vi "ColorDetect3.0_Display.vi"(4 "Fine Tune Upper":i32(slide)=119 scale=91.0..131.0, 5 "Max_radius":i32(slide)=50 scale=0.0..100.0, 6 "Fine Tune  Lower":i32(slide)=98 scale=85.0..125.0, 7 "Min_radius":i32(slide)=7 scale=0.0..100.0, 8 "error in (no error)":errorcluster, 10 "Upper (SV)":i32(slide)=223 scale=0.0..255.0, 11 "Lower (SV)":i32(slide)=58 scale=0.0..255.0) -> (0 "error out":errorcluster, 2 "XYR found":u32[][](array[numeric])=[[183, 192, 10]], 3 "found":i32=1)   [LabVIEW 2014, in "QwaveSys Raspberry Pi Library.lvlib"]
uses:
  QwaveSys Raspberry Pi Library.lvlib
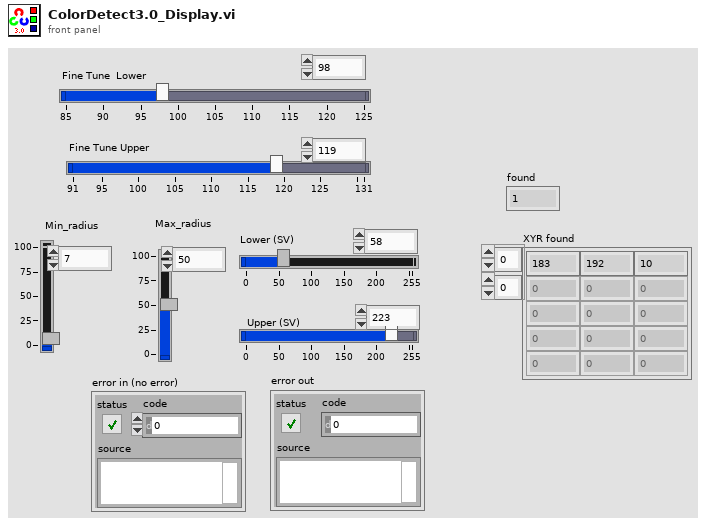
[diagram p1: front panel]
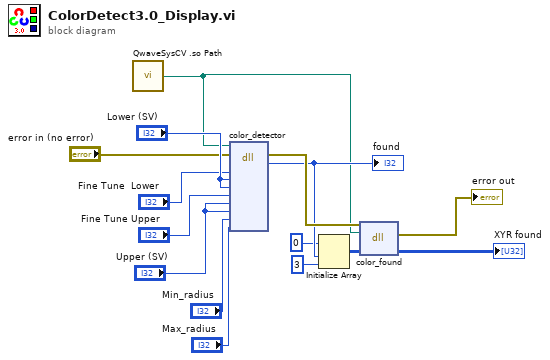
[diagram p0: block diagram]
diagram:
  n1 = call "QwaveSysCV .so Path.vi"() -> ("QwaveSys .so Path"=w5:path)  [unwired: 5 in]
  n2 = dll-call lib="libqwavesys.so" fn="color_detector"(path in=w5, error in="error in (no error)", "lower_h"="Fine Tune  Lower", "lower_s"="Lower (SV)", "lower_v"="Lower (SV)", "upper_h"="Fine Tune Upper", "upper_s"="Upper (SV)", "upper_v"="Upper (SV)", "min_radius"="Min_radius", "max_radius"="Max_radius") -> (error out=w13:errorcluster, "return type"=w11:i32)  [unwired: 9 in, 1 out]
  "found" <- w11
  n3 = Initialize Array "Initialize Array"(u32 0 ("element"), w11, 3 ("dimension size")) -> (w10:u32[][])
  n4 = dll-call lib="libqwavesys.so" fn="color_found"(path in=w5, error in=w13, "found"=w10) -> (error out=→"error out":errorcluster, "found"=→"XYR found":u32[][])  [unwired: 2 in, 1 out]
